vi "LinkedIn OAuth Test.vi"() -> ()   [LabVIEW 2020]
uses:
  Oauth2.LinkedIn/Oauth2.LinkedIn.lvclass
  C:/Data/1_Projects/CIGH_Oauth2/source/Oauth2/Oauth2.lvclass
  Oauth2/Oauth2.lvclass
  <vilib>/LabVIEW Open Source Project/OpenURI/uri/URI.lvclass
  <vilib>/httpClient/LabVIEWHTTPClient.lvlib
panel:
  out "LinkedIn":string
  out "HTTP Response Headers":string
  in  "Client Secret":string
  in  "Client ID":string
  out "LinkedIn Access Token":string
  out "error out":errorcluster
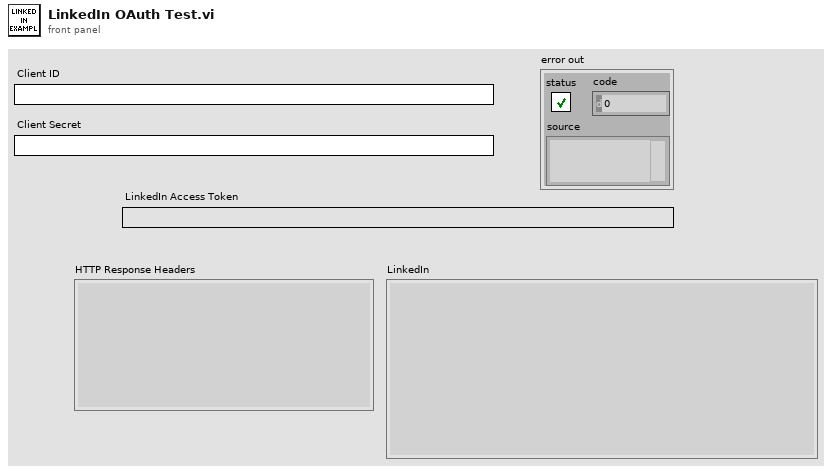
[diagram p1: front panel]
types:
  T1 = typedef "LabVIEWHTTPClient.lvlib/ClientHandle.ctl" = refnum<k1>
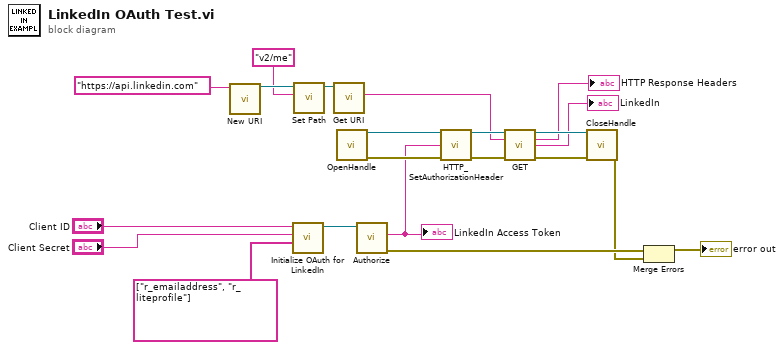
[diagram p0: block diagram]
diagram:
  n1 = call <vilib>:"New URI.vi"("URI"="https://api.linkedin.com" ("path")) -> ("URI"=w21:refnum<class "URI.lvclass">)  [unwired: 9 in, 1 out]
  n2 = call "Initialize OAuth for LinkedIn.vi"("Scopes"=string[] ["r_emailaddress", "r_liteprofile"], "Client Secret"="Client Secret", "Client ID"="Client ID") -> ("Oauth2.LinkedIn"=w1:refnum<class "Oauth2.LinkedIn.lvclass">)  [unwired: 8 in]
  n3 = call <vilib>:"Set Path.vi"("path"="v2/me", "URI in"=w21) -> ("URI out"=w19:refnum<class "URI.lvclass">)  [unwired: 8 in, 1 out]
  n4 = call <vilib>:"Get URI.vi"("URI in"=w19) -> ("URI String"=w12:string)  [unwired: 8 in, 2 out]
  n5 = call <vilib>:"OpenHandle.vi"() -> ("client handle out"=w18:T1, "error out"=w17:errorcluster)  [unwired: 14 in]
  n6 = call "Authorize.vi"("Oauth2 in"=w1) -> ("error out"=w7:errorcluster, "Access Token"=w9:string)  [unwired: 8 in, 1 out]
  "LinkedIn Access Token" <- w9
  n7 = call "HTTP_SetAuthorizationHeader.vi"("Client Handle"=w18, "Access Token"=w9, "error in (no error)"=w17) -> ("client handle dup"=w16:T1, "error out"=w15:errorcluster)  [unwired: 11 in]
  n8 = call <vilib>:"GET.vi"("client handle"=w16, "url"=w12, "error in (no error)"=w15) -> ("client handle out"=w14:T1, "headers"=→"HTTP Response Headers":string, "body"=→"LinkedIn":string, "error out"=w13:errorcluster)  [unwired: 9 in]
  n9 = call <vilib>:"CloseHandle.vi"("client handle"=w14, "error in (no error)"=w13) -> ("error out"=w5:errorcluster)  [unwired: 13 in]
  n10 = Merge Errors(w7, w5) -> (→"error out":errorcluster)
